vi "test_pubsub.vi"() -> ()   [LabVIEW 2019]
panel:
  out "equal send":bool
  out "equal receive":bool
  in  "npub":i32=3
  in  "nsub":i32=2
  out "success?":bool
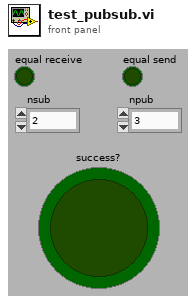
[diagram p1: front panel]
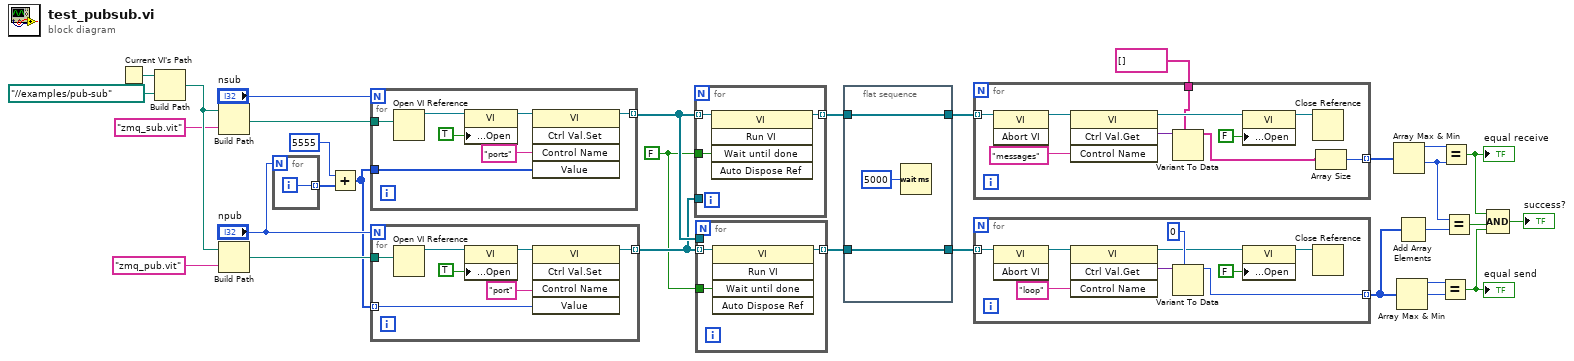
[diagram p0: block diagram]
diagram:
  w17 = FALSE
  n1 = Current VI's Path() -> (path=w5:path)
  n2 = Build Path(base path=w5, name or relative path=path "../../examples/pub-sub" ("VI Path")) -> (appended path=w3:path)
  n3 = Build Path(base path=w3, name or relative path="zmq_sub.vit") -> (appended path=w31:path)
  n4 = Build Path(base path=w3, name or relative path="zmq_pub.vit") -> (appended path=w29:path)
  n5 = for {
    N: "npub" -> [_]
    tunnel: [w32] -> w24 mode=indexing
    i -> [w32]
  }
  n6 = Add(x=5555, y=w24) -> (x+y=w22:i32[])
  n7 = for {
    N: "nsub" -> [_]
    tunnel: [w33] -> w19 mode=indexing
    tunnel: w31 -> [w37]
    tunnel: w22 -> [w35]
    n8 = Open VI Reference(vi path=w37) -> (vi reference=w39:refnum<vi>)  [unwired: 5 in, 1 out]
    n9 = property class="VI"(reference=w39, "Front Panel.Open"=TRUE ("Front Panel Window:Open")) -> (reference out=w36:refnum<vi>)  [unwired: 1 in, 1 out]
    n10 = invoke class="VI" method="Ctrl Val.Set"(reference=w36, "Control Name"="ports", "Value"=w35) -> (reference out=w33:refnum<vi>)  [unwired: 2 in, 4 out]
  }
  n11 = for {
    N: "npub" -> [_]
    tunnel: [w40] -> w18 mode=indexing
    tunnel: w29 -> [w42]
    tunnel: w22 -> [w41] mode=indexing
    n12 = Open VI Reference(vi path=w42) -> (vi reference=w44:refnum<vi>)  [unwired: 5 in, 1 out]
    n13 = property class="VI"(reference=w44, "Front Panel.Open"=TRUE ("Front Panel Window:Open")) -> (reference out=w45:refnum<vi>)  [unwired: 1 in, 1 out]
    n14 = invoke class="VI" method="Ctrl Val.Set"(reference=w45, "Control Name"="port", "Value"=w41) -> (reference out=w40:refnum<vi>)  [unwired: 2 in, 4 out]
  }
  n15 = for {
    tunnel: [w49] -> w21 mode=indexing
    tunnel: w19 -> [w48] mode=indexing
    tunnel: w18 -> [_]
    tunnel: w17 -> [w47]
    n16 = invoke class="VI" method="Run VI"(reference=w48, "Wait until done"=w47) -> (reference out=w49:refnum<vi>)  [unwired: 3 in, 4 out]
  }
  n17 = for {
    tunnel: [w52] -> w20 mode=indexing
    tunnel: w18 -> [w51] mode=indexing
    tunnel: w19 -> [_]
    tunnel: w17 -> [w50]
    n18 = invoke class="VI" method="Run VI"(reference=w51, "Wait until done"=w50) -> (reference out=w52:refnum<vi>)  [unwired: 3 in, 4 out]
  }
  n19 = flat-sequence {
    tunnel: w20 -> [w54]
    tunnel: w21 -> [w53]
    tunnel: [w54] -> w30
    tunnel: [w53] -> w28
    frame #0 {
      n20 = Wait (ms)(milliseconds to wait=u32 5000) -> ()  [unwired: 1 out]
    }
  }
  n21 = for {
    tunnel: w28 -> [w65] mode=indexing
    tunnel: string[] [] -> [w58]
    tunnel: [w56] -> w16 mode=indexing
    n22 = invoke class="VI" method="Abort VI"(reference=w65) -> (reference out=w64:refnum<vi>)  [unwired: 2 in, 2 out]
    n23 = invoke class="VI" method="Ctrl Val.Get"(reference=w64, "Control Name"="messages") -> (reference out=w60:refnum<vi>, "Get Control Value Variant"=w62:variant)  [unwired: 2 in, 2 out]
    n24 = Variant To Data(type=w58, Variant=w62) -> (data=w57:string[])  [unwired: 1 in, 1 out]
    n25 = property class="VI"(reference=w60, "Front Panel.Open"=FALSE ("Front Panel Window:Open")) -> (reference out=w61:refnum<vi>)  [unwired: 1 in, 1 out]
    n26 = Close Reference(reference=w61) -> ()  [unwired: 1 in, 1 out]
    n27 = Array Size(array=w57) -> (size(s)=w56:i32)
  }
  n28 = for {
    tunnel: w30 -> [w74] mode=indexing
    tunnel: [w66] -> w7 mode=indexing
    n29 = invoke class="VI" method="Abort VI"(reference=w74) -> (reference out=w73:refnum<vi>)  [unwired: 2 in, 2 out]
    n30 = invoke class="VI" method="Ctrl Val.Get"(reference=w73, "Control Name"="loop") -> (reference out=w68:refnum<vi>, "Get Control Value Variant"=w71:variant)  [unwired: 2 in, 2 out]
    n31 = Variant To Data(type=0, Variant=w71) -> (data=w66:i32)  [unwired: 1 in, 1 out]
    n32 = property class="VI"(reference=w68, "Front Panel.Open"=FALSE ("Front Panel Window:Open")) -> (reference out=w69:refnum<vi>)  [unwired: 1 in, 1 out]
    n33 = Close Reference(reference=w69) -> ()  [unwired: 1 in, 1 out]
  }
  n34 = Array Max & Min(array=w16) -> (max value=w15:i32, min value=w13:i32)  [unwired: 2 out]
  n35 = Array Max & Min(array=w7) -> (max value=w12:i32, min value=w14:i32)  [unwired: 2 out]
  n36 = Add Array Elements(numeric array=w7) -> (sum=w6:i32)
  n37 = Equal?(x=w12, y=w14) -> (x = y?=w11:bool)
  "equal send" <- w11
  n38 = Equal?(x=w15, y=w13) -> (x = y?=w9:bool)
  "equal receive" <- w9
  n39 = Equal?(x=w13, y=w6) -> (x = y?=w10:bool)
  n40 = Compound Arithmetic op=AND(w9, w10, w11) -> (→"success?":bool)
